vi "calcFFTfreqArray_Ch3.vi"(2 "N Freqs.":i32=32, 3 "Freq. Step (Hz)":dbl=12.0 format="%.2f") -> (1 "Array":dbl[](array[numeric])=[0.0, 12.0, 24.0, 36.0, 48.0, 60.0, 72.0, 84.0, 96.0, 108.0, 120.0, 132.0, 144.0, 156.0, 168.0, 180.0, 192.0, 204.0, 216.0, 228.0, 240.0, 252.0, 264.0, 276.0, 288.0, 300.0, 312.0, 324.0, 336.0, 348.0, 360.0, 372.0] format="%.1f")   [LabVIEW 2015]
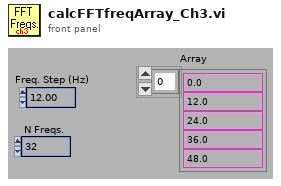
[diagram p1: front panel]
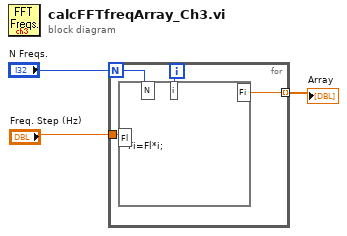
[diagram p0: block diagram]
diagram:
  n1 = for {
    N: "N Freqs." -> [w7]
    tunnel: "Freq. Step (Hz)" -> [w6]
    tunnel: [w4] -> w1 mode=indexing
    i -> [w5]
    # "Calculate Frequency"
    n2 = formula code="Fi=Fl*i;"("N"=w7, "Fl"=w6, "i"=w5) -> ("Fi"=w4:dbl)
  }
  "Array" <- w1
